vi "factoriel.vi"() -> ()   [LabVIEW 2014]
panel:
  out "Resultat":dbl
  out "indice de la boucle":dbl
  in  "Factoriel n":dbl
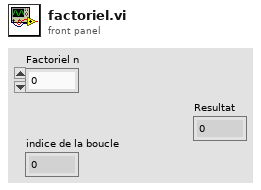
[diagram p1: front panel]
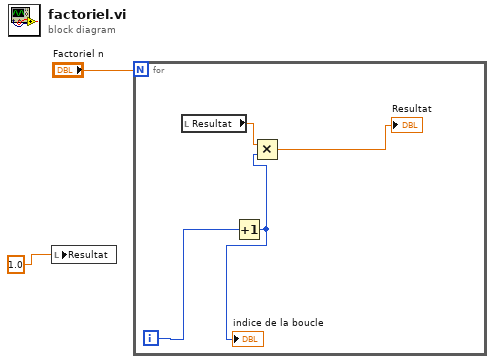
[diagram p0: block diagram]
diagram:
  n1 = local write "Resultat"(1.0) -> ()
  n2 = for {
    N: "Factoriel n" -> [_]
    i -> [w5]
    n3 = local read "Resultat"() -> (w6:dbl)
    n4 = Increment(x=w5) -> (x+1=w3:i32)
    "indice de la boucle" <- w3
    n5 = Multiply(x=w6, y=w3) -> (x*y=→"Resultat":dbl)
  }
